vi "Modify Nodes and Edges.vi"(11 "Graph in":refnum<class "Graph.lvclass">) -> (3 "Graphviz out":refnum<class "Graphviz.lvclass">)   [LabVIEW 2020, in "SimpleDependencyInspector.lvlib"]
uses:
  SimpleDependencyInspector.lvlib
  <vilib>/GraphBuilder/Graph/Graph.lvclass
  <vilib>/GraphBuilder/Renderer/Graphviz/Graphviz.lvclass
  <vilib>/GraphBuilder/Renderer/Graphviz/Graph Direction.ctl
  <vilib>/GraphBuilder/Renderer/Graphviz/Specific Edge Shape Def.ctl
  <vilib>/GraphBuilder/Shapes/Edge/Graphviz/Graphviz Edge Shape.lvclass
  <vilib>/GraphBuilder/Edge/Edge.lvclass
  <vilib>/GraphBuilder/Shapes/Edge/Graphviz/Shape.ctl
  <vilib>/GraphBuilder/Shapes/Edge/Graphviz/Style.ctl
  <vilib>/GraphBuilder/Shapes/Node/Graphviz/Graphviz Node Shape.lvclass
  <vilib>/GraphBuilder/Renderer/Graphviz/Specific Node Shape Def.ctl
  <vilib>/GraphBuilder/Node/Node.lvclass
  <vilib>/GraphBuilder/Shapes/Node/Graphviz/Shape.ctl
  <vilib>/GraphBuilder/Shapes/Node/Graphviz/Colors.ctl
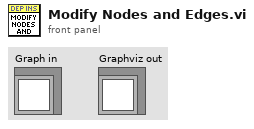
[diagram p1: front panel]
types:
  T1 = typedef "GraphBuilder.lvlib/Graphviz.lvclass/Graph Direction.ctl" = enum16{"Top to Bottom", "Left To Right", "Bottom to Top", "Right to Left"}
  T2 = typedef "GraphBuilder.lvlib/Graphviz.lvclass/Specific Node Shape Def.ctl" = cluster{"Graphviz Node Shape":refnum<class "Graphviz Node Shape.lvclass">, "Node":refnum<class "Node.lvclass">}
  T3 = typedef "GraphBuilder.lvlib/Graphviz Node Shape.lvclass/Colors.ctl" = enum16{"aliceblue", "antiquewhite", "aqua", "aquamarine", "azure", "beige", "bisque", "black", "blanchedalmond", "blue", "blueviolet", "brown", "burlywood", "cadetblue", "chartreuse", "chocolate", "coral", "cornflowerblue", "cornsilk", "crimson", "cyan", "darkblue", "darkcyan", "darkgoldenrod", "darkgray", "darkgreen", "darkgrey", "darkkhaki", "darkmagenta", "darkolivegreen", "darkorange", "darkorchid", "darkred", "darksalmon", "darkseagreen", "darkslateblue", "darkslategray", "darkslategrey", "darkturquoise", "darkviolet", "deeppink", "deepskyblue", "dimgray", "dimgrey", "dodgerblue", "firebrick", "floralwhite", "forestgreen", "fuchsia", "gainsboro", "ghostwhite", "gold", "goldenrod", "gray", "green", "greenyellow", "grey", "honeydew", "hotpink", "indianred", "indigo", "ivory", "khaki", "lavender", "lavenderblush", "lawngreen", "lemonchiffon", "lightblue", "lightcoral", "lightcyan", "lightgoldenrodyellow", "lightgray", "lightgreen", "lightgrey", "lightpink", "lightsalmon", "lightseagreen", "lightskyblue", "lightslategray", "lightslategrey", "lightsteelblue", "lightyellow", "lime", "limegreen", "linen", "magenta", "maroon", "mediumaquamarine", "mediumblue", "mediumorchid", "mediumpurple", "mediumseagreen", "mediumslateblue", "mediumspringgreen", "mediumturquoise", "mediumvioletred", "midnightblue", "mintcream", "mistyrose", "moccasin", "navajowhite", "navy", "oldlace", "olive", "olivedrab", "orange", "orangered", "orchid", "palegoldenrod", "palegreen", "paleturquoise", "palevioletred", "papayawhip", "peachpuff", "peru", "pink", "plum", "powderblue", "purple", "red", "rosybrown", "royalblue", "saddlebrown", "salmon", "sandybrown", "seagreen", "seashell", "sienna", "silver", "skyblue", "slateblue", "slategray", "slategrey", "snow", "springgreen", "steelblue", "tan", "teal", "thistle", "tomato", "turquoise", "violet", "wheat", "white", "whitesmoke", "yellow", "yellowgreen"}
  T4 = typedef "GraphBuilder.lvlib/Graphviz Node Shape.lvclass/Shape.ctl" = enum16{"box", "polygon", "ellipse", "oval", "circle", "point", "egg", "triangle", "plaintext", "plain", "diamond", "trapezium", "parallelogram", "house", "pentagon", "hexagon", "septagon", "octagon", "doublecircle", "doubleoctagon", "tripleoctagon", "invtriangle", "invtrapezium", "invhouse", "Mdiamond", "Msquare", "Mcircle", "rect", "rectangle", "square", "star", "none", "underline", "cylinder", "note", "tab", "folder", "box3D", "component", "promoter", "cds", "terminator", "utr", "primersite", "restrictionsite", "fivepoverhang", "threepoverhang", "noverhang", "assembly", "signature", "insulator", "ribosite", "rnastab", "proteasesite", "proteinstab", "rpromoter", "rarrow", "larrow", "lpromoter"}
  T5 = typedef "GraphBuilder.lvlib/Graphviz Edge Shape.lvclass/Style.ctl" = enum8{"filled", "invisible", "diagonals", "rounded", "dashed", "dotted", "solid", "bold"}
  T6 = typedef "GraphBuilder.lvlib/Graphviz Edge Shape.lvclass/Shape.ctl" = enum16{"box", "lbox", "rbox", "obox", "olbox", "orbox", "crow", "lcrow", "rcrow", "diamond", "ldiamond", "rdiamond", "odiamond", "oldiamond", "ordiamond", "dot", "odot", "inv", "linv", "rinv", "oinv", "olinv", "orinv", "none", "normal", "lnormal", "rnormal", "onormal", "olnormal", "ornormal", "tee", "ltee", "rtee", "vee", "lvee", "rvee", "curve", "lcurve", "rcurve", "icurve", "licurve", "ricurve"}
  T7 = typedef "GraphBuilder.lvlib/Graphviz.lvclass/Specific Edge Shape Def.ctl" = cluster{"Graphviz Edge Shape":refnum<class "Graphviz Edge Shape.lvclass">, "Edge":refnum<class "Edge.lvclass">}
  T8 = typedef "GraphBuilder.lvlib/Graphviz Edge Shape.lvclass/Colors.ctl" = enum16{"aliceblue", "antiquewhite", "aqua", "aquamarine", "azure", "beige", "bisque", "black", "blanchedalmond", "blue", "blueviolet", "brown", "burlywood", "cadetblue", "chartreuse", "chocolate", "coral", "cornflowerblue", "cornsilk", "crimson", "cyan", "darkblue", "darkcyan", "darkgoldenrod", "darkgray", "darkgreen", "darkgrey", "darkkhaki", "darkmagenta", "darkolivegreen", "darkorange", "darkorchid", "darkred", "darksalmon", "darkseagreen", "darkslateblue", "darkslategray", "darkslategrey", "darkturquoise", "darkviolet", "deeppink", "deepskyblue", "dimgray", "dimgrey", "dodgerblue", "firebrick", "floralwhite", "forestgreen", "fuchsia", "gainsboro", "ghostwhite", "gold", "goldenrod", "gray", "green", "greenyellow", "grey", "honeydew", "hotpink", "indianred", "indigo", "ivory", "khaki", "lavender", "lavenderblush", "lawngreen", "lemonchiffon", "lightblue", "lightcoral", "lightcyan", "lightgoldenrodyellow", "lightgray", "lightgreen", "lightgrey", "lightpink", "lightsalmon", "lightseagreen", "lightskyblue", "lightslategray", "lightslategrey", "lightsteelblue", "lightyellow", "lime", "limegreen", "linen", "magenta", "maroon", "mediumaquamarine", "mediumblue", "mediumorchid", "mediumpurple", "mediumseagreen", "mediumslateblue", "mediumspringgreen", "mediumturquoise", "mediumvioletred", "midnightblue", "mintcream", "mistyrose", "moccasin", "navajowhite", "navy", "oldlace", "olive", "olivedrab", "orange", "orangered", "orchid", "palegoldenrod", "palegreen", "paleturquoise", "palevioletred", "papayawhip", "peachpuff", "peru", "pink", "plum", "powderblue", "purple", "red", "rosybrown", "royalblue", "saddlebrown", "salmon", "sandybrown", "seagreen", "seashell", "sienna", "silver", "skyblue", "slateblue", "slategray", "slategrey", "snow", "springgreen", "steelblue", "tan", "teal", "thistle", "tomato", "turquoise", "violet", "wheat", "white", "whitesmoke", "yellow", "yellowgreen"}
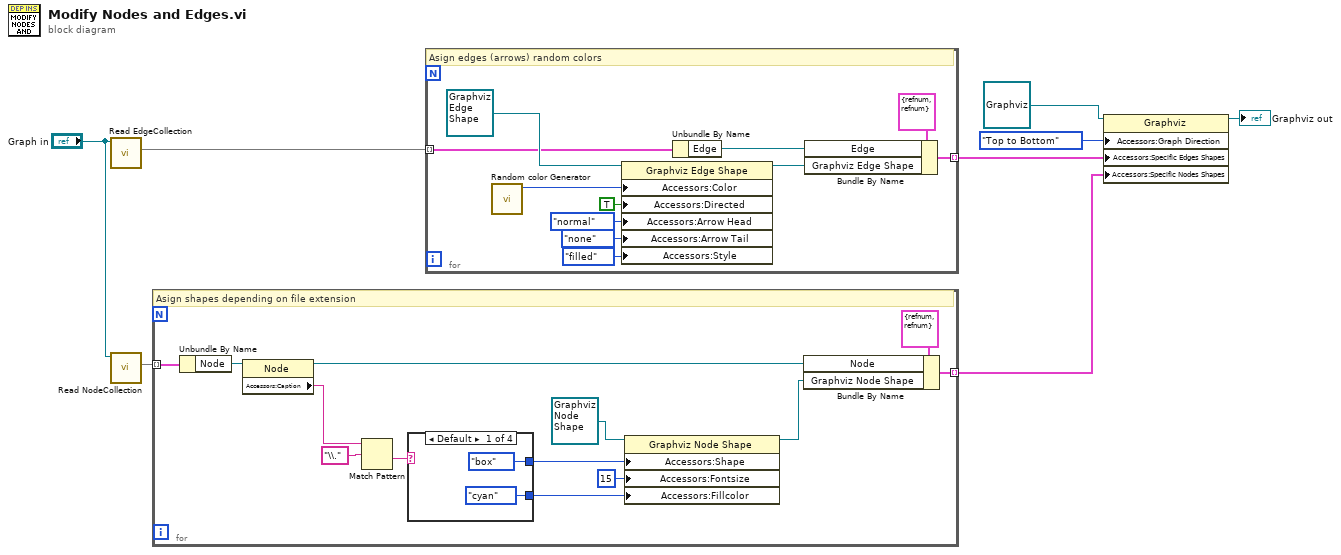
[diagram p0: block diagram]
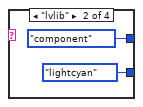
[diagram p2: hidden frame]
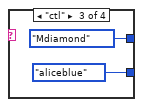
[diagram p3: hidden frame]
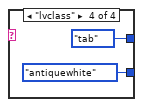
[diagram p4: hidden frame]
diagram:
  n1 = call-dynamic "Read EdgeCollection.vi"("Graph in"="Graph in") -> ("EdgeCollection"=w7:map{string, refnum<class "Edge.lvclass">})  [unwired: 9 in, 1 out]
  n2 = call-dynamic "Read NodeCollection.vi"("Graph in"="Graph in") -> ("NodeCollection"=w2:map{string, refnum<class "Node.lvclass">})  [unwired: 9 in, 1 out]
  n3 = for {
    tunnel: w2 -> [w21] mode=indexing
    tunnel: [w15] -> w3 mode=indexing
    # "Asign shapes depending on file extension"
    n4 = Unbundle By Name(w21) -> ("Node"=w20:refnum<class "Node.lvclass">)
    n5 = property class="Node"(reference=w20) -> (reference out=w16:refnum<class "Node.lvclass">, "Accessors:Caption"=w14:string)  [unwired: 1 in, 1 out]
    n6 = Match Pattern(string=w14, regular expression="\\.") -> (after substring=w12:string)  [unwired: 1 in, 3 out]
    n7 = case shown="Default" w12 {
      tunnel: [Shape."box" ("Shape") Shape."component" ("Shape") Shape."Mdiamond" ("Shape") Shape."tab" ("Shape")] -> w11
      tunnel: [Colors."cyan" ("Fillcolor") Colors."lightcyan" ("Fillcolor") Colors."aliceblue" ("Fillcolor") Colors."antiquewhite" ("Fillcolor")] -> w9
      frame Default {
      }
      frame "lvlib" {
      }
      frame "ctl" {
      }
      frame "lvclass" {
      }
    }
    n8 = property class="Graphviz Node Shape"(reference=refnum<class "Graphviz Node Shape.lvclass"> refnum ("Graphviz Node Shape"), "Accessors:Shape"=w11, "Accessors:Fontsize"=u8 15 ("Fontsize"), "Accessors:Fillcolor"=w9) -> (reference out=w18:refnum<class "Graphviz Node Shape.lvclass">)  [unwired: 1 in, 1 out]
    n9 = Bundle By Name(cluster=T2 {"Graphviz Node Shape"=refnum, "Node"=refnum} ("Specific Node Shape"), "Node"=w16, "Graphviz Node Shape"=w18) -> (w15:T2)
  }
  n10 = for {
    tunnel: w7 -> [w34] mode=indexing
    tunnel: [w32] -> w8 mode=indexing
    # "Asign edges (arrows) random colors"
    n11 = call "Random color Generator.vi"() -> ("Random Color"=w31:T8)  [unwired: 11 in]
    n12 = property class="Graphviz Edge Shape"(reference=refnum<class "Graphviz Edge Shape.lvclass"> refnum ("GraphBuilder.lvlib:Graphviz Edge Shape.lvclass"), "Accessors:Color"=w31, "Accessors:Directed"=TRUE ("Directed"), "Accessors:Arrow Head"=Shape."normal" ("Arrow Head"), "Accessors:Arrow Tail"=Shape."none" ("Arrow Tail"), "Accessors:Style"=Style."filled" ("Style")) -> (reference out=w36:refnum<class "Graphviz Edge Shape.lvclass">)  [unwired: 1 in, 1 out]
    n13 = Unbundle By Name(w34) -> ("Edge"=w33:refnum<class "Edge.lvclass">)
    n14 = Bundle By Name(cluster=T7 {"Graphviz Edge Shape"=refnum, "Edge"=refnum} ("Specific Node Shape"), "Edge"=w33, "Graphviz Edge Shape"=w36) -> (w32:T7)
  }
  n15 = property class="Graphviz"(reference=refnum<class "Graphviz.lvclass"> refnum ("GraphBuilder.lvlib:Graphviz.lvclass"), "Accessors:Graph Direction"=Graph_Direction."Top to Bottom" ("Graph Direction"), "Accessors:Specific Edges Shapes"=w8, "Accessors:Specific Nodes Shapes"=w3) -> (reference out=→"Graphviz out":refnum<class "Graphviz.lvclass">)  [unwired: 1 in, 1 out]
